vi "癌变与普通病变选择界面.vi"() -> ()   [LabVIEW 2018]
panel:
  in  "早癌EGC按钮":bool
  in  "癌前病变按钮":bool
  # "诊\n断\n系\n统\n选\n择"
  # "癌前病变诊断系统"
  # "早癌EGC诊断系统"
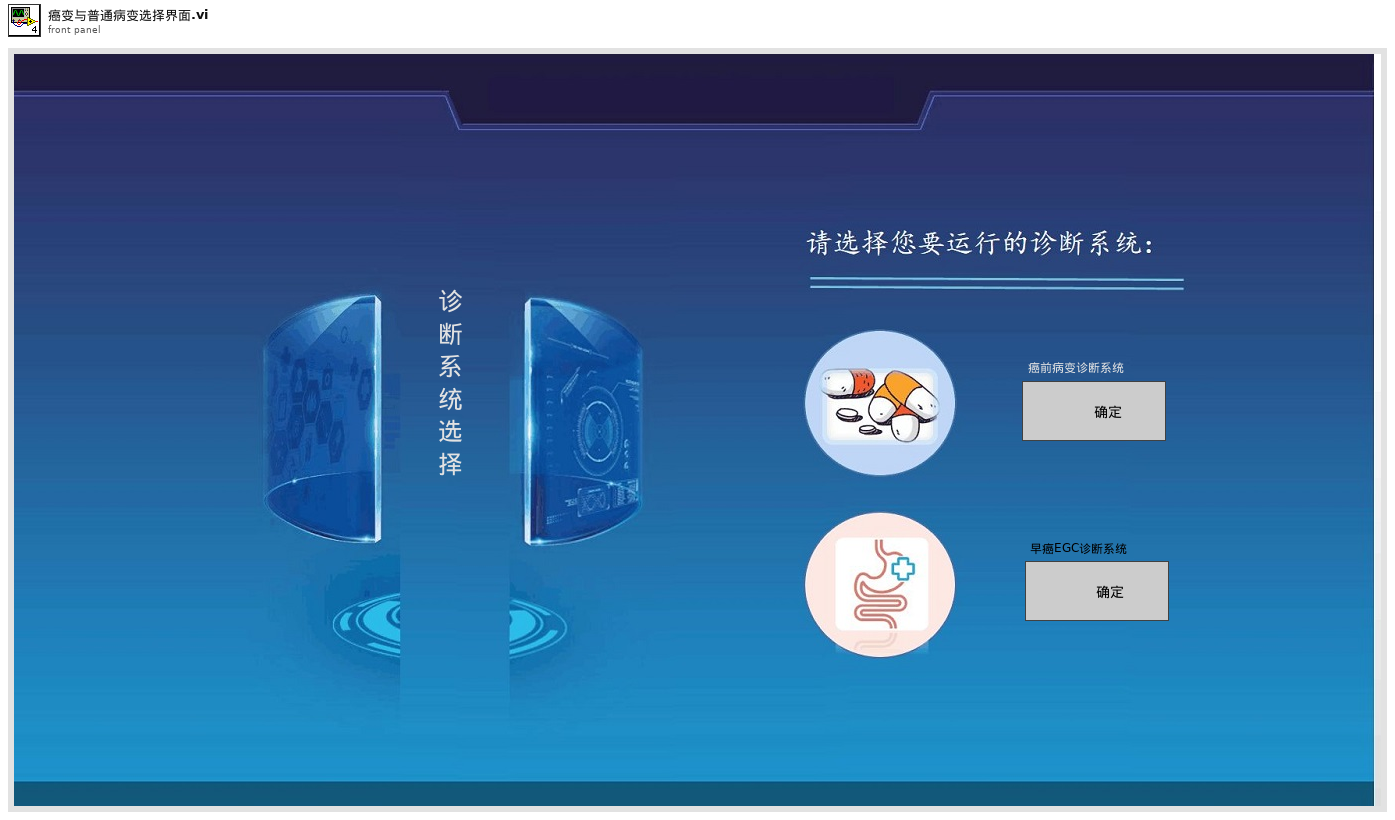
[diagram p1: front panel]
types:
  T1 = enum32{"Invalid", "Standard", "Closed", "Hidden", "Minimized", "Maximized"}
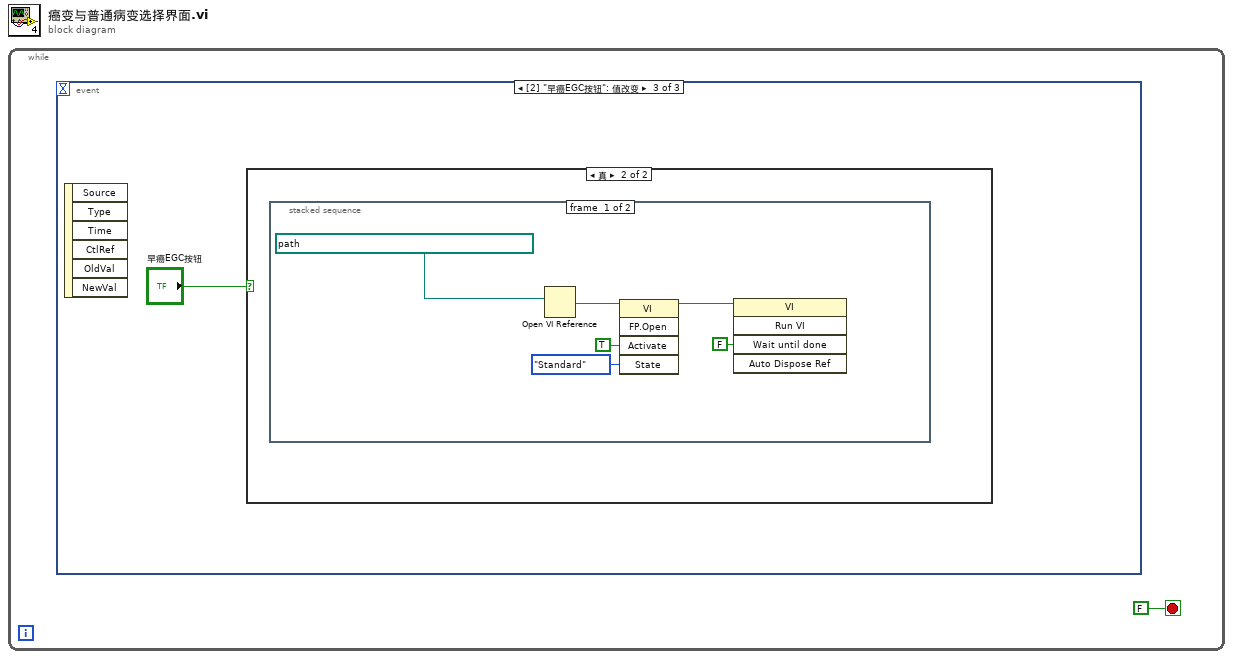
[diagram p0: block diagram]
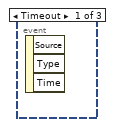
[diagram p2: hidden frame]
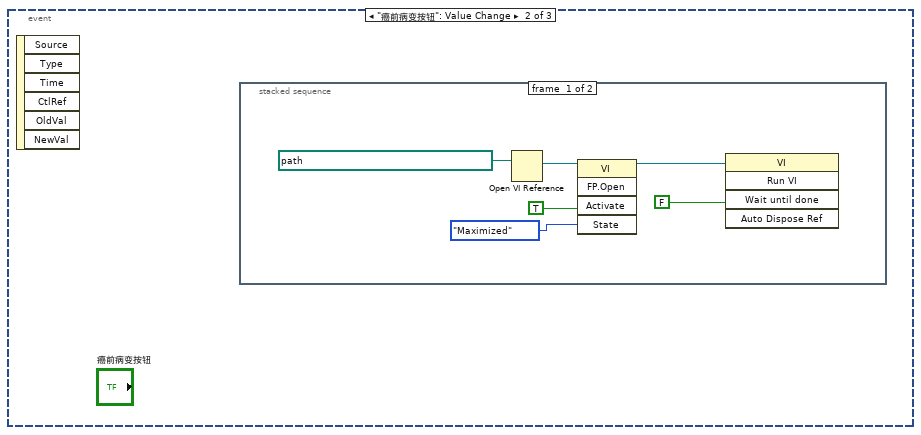
[diagram p3: hidden frame]
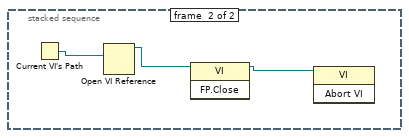
[diagram p4: hidden frame]
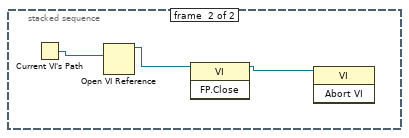
[diagram p6: hidden frame]
diagram:
  n1 = while {
    stop <- FALSE stop-if-true
    n2 = event shown="[2] \"早癌EGC按钮\": 值改变" {
      selector: _ -> [_ _ _]
      dyn-events: _ -> [_ _ _]
      timeout: _ -> [_ _ _]
      event Timeout {
        n3 = event-data() -> ()  [unwired: 1 in, 3 out]
      }
      event "癌前病变按钮": Value Change {
        n4 = event-data() -> ()  [unwired: 1 in, 6 out]
        n5 = stacked-sequence {
          frame #0 {
            n6 = Open VI Reference(vi path=path "E:/登陆系统重写/病人基本信息编辑.vi" ("VI路径")) -> (vi reference=w6:refnum<vi>)  [unwired: 5 in, 1 out]
            n7 = invoke class="VI" method="FP.Open"(reference=w6, "Activate"=TRUE ("激活？"), "State"=T1."Maximized" ("状态")) -> (reference out=w7:refnum<vi>)  [unwired: 2 in, 4 out]
            n8 = invoke class="VI" method="Run VI"(reference=w7, "Wait until done"=FALSE ("结束前等待")) -> ()  [unwired: 3 in, 5 out]
          }
          frame #1 {
            n9 = Current VI's Path() -> (path=w10:path)
            n10 = Open VI Reference(vi path=w10) -> (vi reference=w9:refnum<vi>)  [unwired: 5 in, 1 out]
            n11 = invoke class="VI" method="FP.Close"(reference=w9) -> (reference out=w8:refnum<vi>)  [unwired: 2 in, 2 out]
            n12 = invoke class="VI" method="Abort VI"(reference=w8) -> ()  [unwired: 2 in, 3 out]
          }
        }
      }
      event "早癌EGC按钮": Value Change {
        n13 = event-data() -> ()  [unwired: 1 in, 6 out]
        n14 = case shown="真" "早癌EGC按钮" {
          frame False {
          }
          frame True {
            n15 = stacked-sequence {
              frame #0 {
                n16 = Open VI Reference(vi path=path "E:/登陆系统重写/病人基本信息编辑 (早癌）.vi" ("VI路径")) -> (vi reference=w17:refnum<vi>)  [unwired: 5 in, 1 out]
                n17 = invoke class="VI" method="FP.Open"(reference=w17, "Activate"=TRUE ("激活？"), "State"=T1."Standard" ("状态")) -> (reference out=w16:refnum<vi>)  [unwired: 2 in, 4 out]
                n18 = invoke class="VI" method="Run VI"(reference=w16, "Wait until done"=FALSE ("结束前等待")) -> ()  [unwired: 3 in, 5 out]
              }
              frame #1 {
                n19 = Current VI's Path() -> (path=w20:path)
                n20 = Open VI Reference(vi path=w20) -> (vi reference=w19:refnum<vi>)  [unwired: 5 in, 1 out]
                n21 = invoke class="VI" method="FP.Close"(reference=w19) -> (reference out=w18:refnum<vi>)  [unwired: 2 in, 2 out]
                n22 = invoke class="VI" method="Abort VI"(reference=w18) -> ()  [unwired: 2 in, 3 out]
              }
            }
          }
        }
      }
    }
  }
